vi "ShiftRegister_2.vi"() -> ()   [LabVIEW 2023]
panel:
  out "Numeric 2":dbl
  out "Numeric":dbl
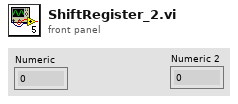
[diagram p1: front panel]
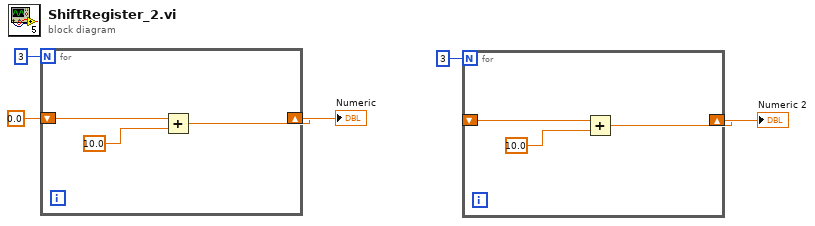
[diagram p0: block diagram]
diagram:
  n1 = for {
    N: 3 -> [_]
    shift-right: [w6] -> w4
    shift-left: 0.0 -> [w8]
    n2 = Add(x=w8, y=10.0) -> (x+y=w6:dbl)
  }
  "Numeric" <- w4
  n3 = for {
    N: 3 -> [_]
    shift-right: [w9] -> w2
    shift-left: _ -> [w11]
    n4 = Add(x=w11, y=10.0) -> (x+y=w9:dbl)
  }
  "Numeric 2" <- w2
